vi "Send Starter Kit Message.vi"(8 "error in (no error)":errorcluster, 10 "message":T1={"message type"=enum."Motor Vel SP", "message data"=variant}, 11 "connection ID in":refnum<k5>) -> (0 "error out":errorcluster, 3 "connection ID out":refnum<k5>)   [LabVIEW 2010]
uses:
  Starter Kit Message.ctl
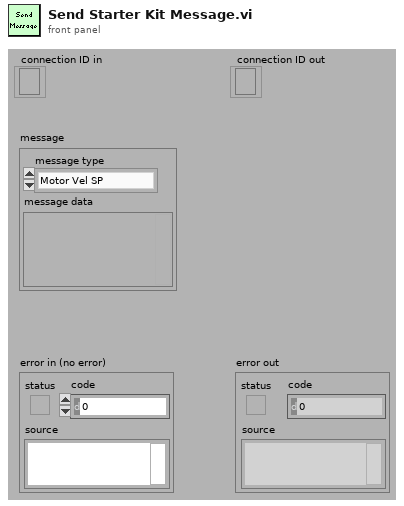
[diagram p1: front panel]
types:
  T1 = typedef "Starter Kit Message.ctl" = cluster{"message type":enum16{"Heartbeat", "Motor Vel SP", "Servo Angle", "Stop"}, "message data":variant}
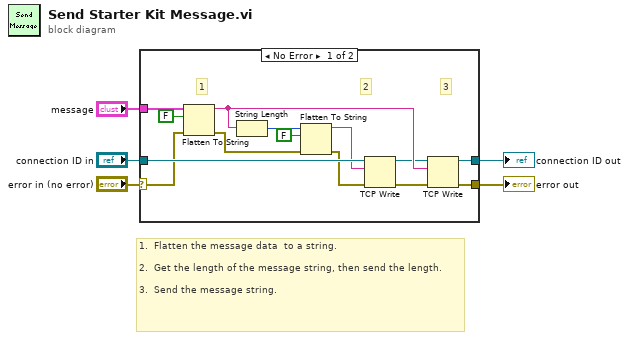
[diagram p0: block diagram]
diagram:
  # "1.  Flatten the message data  to a string.\n\n2.  Get the length of the message string, then send the length.\n\n3.  Send the message string."
  n1 = case shown="No Error" "error in (no error)" {
    selector: "error in (no error)" -> [w6 w20]
    tunnel: "message" -> [w19 _]
    tunnel: [w17 w21] -> w4
    tunnel: [w16 w20] -> w3
    tunnel: "connection ID in" -> [w14 w21]
    frame No Error {
      # "3"
      # "2"
      # "1"
      n2 = Flatten To String(anything=w19, prepend array or string size? (T)=FALSE, error in (no error)=w6) -> (data string=w15:string, error out=w8:errorcluster)  [unwired: 2 out]
      n3 = String Length(string=w15) -> (length=w11:i32)
      n4 = Flatten To String(anything=w11, prepend array or string size? (T)=FALSE, error in (no error)=w8) -> (data string=w9:string, error out=w7:errorcluster)  [unwired: 1 in, 1 out]
      n5 = TCP Write(connection ID=w14, data in=w9, error in (no error)=w7) -> (connection ID out=w13:refnum<k5>, error out=w12:errorcluster)  [unwired: 2 out]
      n6 = TCP Write(connection ID=w13, data in=w15, error in (no error)=w12) -> (connection ID out=w17:refnum<k5>, error out=w16:errorcluster)  [unwired: 2 out]
    }
    frame Error {
    }
  }
  "connection ID out" <- w4
  "error out" <- w3
